vi "InRangePosition.vi"(11 "Input Positions in":i32[][](array[numeric])) -> (3 "Output Positions":i32[][](array[numeric]))   [LabVIEW 2019]
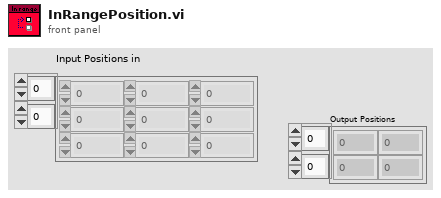
[diagram p1: front panel]
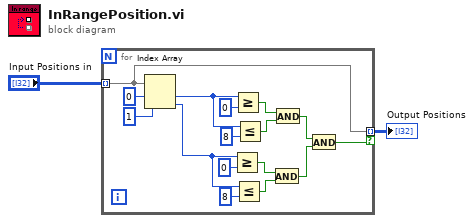
[diagram p0: block diagram]
diagram:
  n1 = for {
    tunnel: "Input Positions in" -> [w4] mode=indexing
    tunnel: [w4] -> w2 mode=indexing if=w3
    n2 = Index Array(array=w4, index #1=0 ("index"), index #2=1 ("index")) -> (element #1=w16:i32, element #2=w7:i32)
    n3 = Greater Or Equal?(x=w7, y=0) -> (x >= y?=w10:bool)
    n4 = Greater Or Equal?(x=w16, y=0) -> (x >= y?=w13:bool)
    n5 = Less Or Equal?(x=w7, y=8) -> (x <= y?=w11:bool)
    n6 = Less Or Equal?(x=w16, y=8) -> (x <= y?=w12:bool)
    n7 = And(x=w10, y=w11) -> (x .and. y?=w6:bool)
    n8 = And(x=w13, y=w12) -> (x .and. y?=w5:bool)
    n9 = And(x=w5, y=w6) -> (x .and. y?=w3:bool)
  }
  "Output Positions" <- w2
